vi "Close_Panel_and_Abort.vi"(1 "Vi path":path, 2 "stop":bool) -> ()   [LabVIEW 2010]
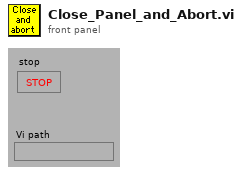
[diagram p1: front panel]
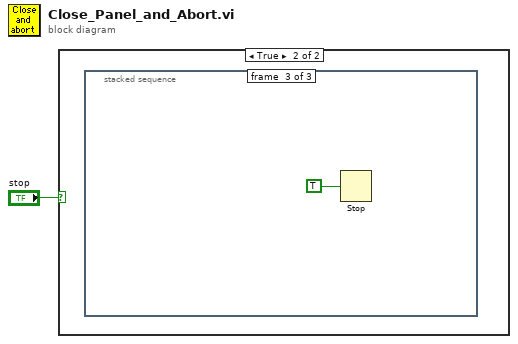
[diagram p0: block diagram]
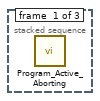
[diagram p3: hidden frame]
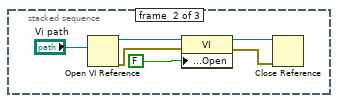
[diagram p4: hidden frame]
diagram:
  n1 = case shown="True" "stop" {
    frame False {
    }
    frame True {
      n2 = stacked-sequence {
        frame #0 {
          n3 = call "Program_Active_Aborting.vi"() -> ()  [unwired: 6 out]
        }
        frame #1 {
          n4 = Open VI Reference(vi path="Vi path") -> (vi reference=w7:refnum<vi>, error out=w3:errorcluster)  [unwired: 1 in, 4 out]
          n5 = property class="VI"(reference=w7, error in=w3, "Front Panel Window:Open"=FALSE) -> (reference out=w5:refnum<vi>, error out=w4:errorcluster)
          n6 = Close Reference(reference=w5, error in (no error)=w4) -> ()  [unwired: 1 out]
        }
        frame #2 {
          n7 = Stop(stop? (T)=TRUE) -> ()
        }
      }
    }
  }
